vi "Calibration.vi"   [LabVIEW 2013]
uses:
  Global Variables.vi
  Global Refnums.vi
types:
  T1 = typedef "WPI_AnalogChannelDevRef.ctl" = cluster{"DevStatus":errorcluster, "Analog Module":T2, "Analog Channel":T3}
  T2 = typedef "FPGA_TypedefAnalogModule.ctl" = enum16{"Analog Module 1", "Analog Module 2"}
  T3 = typedef "FPGA_AIChannel.ctl" = enum8{"AI 1", "AI 2", "AI 3", "AI 4", "AI 5", "AI 6", "AI 7", "AI 8", "Invalid"}
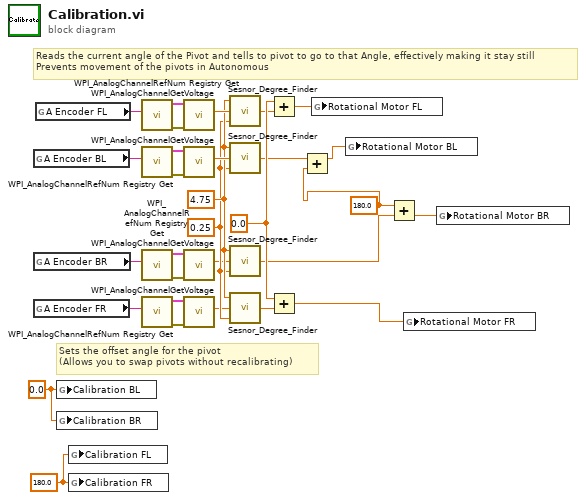
[diagram p0: block diagram]
diagram:
  w1 = 180.0 ("x")
  w22 = 0.0
  w8 = 0.25
  w9 = 4.75
  w29 = 0.0
  w30 = 180.0
  # "Sets the offset angle for the pivot\n(Allows you to swap pivots without recalibrating)"
  # "Reads the current angle of the Pivot and tells to pivot to go to that Angle, effectively making it stay still\nPrevents movement of the pivots in Autonomous"
  n1 = global read "Global Refnums.vi" "A Encoder BL"() -> (w28:string)
  n2 = global read "Global Refnums.vi" "A Encoder BR"() -> (w27:string)
  n3 = global read "Global Refnums.vi" "A Encoder FR"() -> (w25:string)
  n4 = global read "Global Refnums.vi" "A Encoder FL"() -> (w26:string)
  n5 = global write "Global Variables.vi" "Calibration BL"(w29) -> ()
  n6 = global write "Global Variables.vi" "Calibration BR"(w29) -> ()
  n7 = global write "Global Variables.vi" "Calibration FL"(w30) -> ()
  n8 = global write "Global Variables.vi" "Calibration FR"(w30) -> ()
  n9 = call <vilib>:"WPI_AnalogChannelRefNum Registry Get.vi"("refnum name"=w26) -> ("error out"=w17:errorcluster, "AIDeviceRef"=w16:T1)  [unwired: 9 in]
  n10 = call <vilib>:"WPI_AnalogChannelRefNum Registry Get.vi"("refnum name"=w28) -> ("error out"=w20:errorcluster, "AIDeviceRef"=w21:T1)  [unwired: 9 in]
  n11 = call <vilib>:"WPI_AnalogChannelRefNum Registry Get.vi"("refnum name"=w27) -> ("error out"=w19:errorcluster, "AIDeviceRef"=w18:T1)  [unwired: 9 in]
  n12 = call <vilib>:"WPI_AnalogChannelRefNum Registry Get.vi"("refnum name"=w25) -> ("error out"=w15:errorcluster, "AIDeviceRef"=w14:T1)  [unwired: 9 in]
  n13 = call <vilib>:"WPI_AnalogChannelGetVoltage.vi"("error in (no error)"=w17, "AIDeviceRef"=w16) -> ("Voltage"=w12:dbl)  [unwired: 7 in, 2 out]
  n14 = call <vilib>:"WPI_AnalogChannelGetVoltage.vi"("error in (no error)"=w20, "AIDeviceRef"=w21) -> ("Voltage"=w11:dbl)  [unwired: 7 in, 2 out]
  n15 = call <vilib>:"WPI_AnalogChannelGetVoltage.vi"("error in (no error)"=w19, "AIDeviceRef"=w18) -> ("Voltage"=w7:dbl)  [unwired: 7 in, 2 out]
  n16 = call <vilib>:"WPI_AnalogChannelGetVoltage.vi"("error in (no error)"=w15, "AIDeviceRef"=w14) -> ("Voltage"=w6:dbl)  [unwired: 7 in, 2 out]
  n17 = call "Sesnor_Degree_Finder.vi"("Minimum Volts"=w8, "Voltage"=w12, "Max Volts"=w9) -> ("Degrees"=w13:dbl)
  n18 = call "Sesnor_Degree_Finder.vi"("Minimum Volts"=w8, "Voltage"=w11, "Max Volts"=w9) -> ("Degrees"=w10:dbl)
  n19 = call "Sesnor_Degree_Finder.vi"("Minimum Volts"=w8, "Voltage"=w7, "Max Volts"=w9) -> ("Degrees"=w5:dbl)
  n20 = call "Sesnor_Degree_Finder.vi"("Minimum Volts"=w8, "Voltage"=w6, "Max Volts"=w9) -> ("Degrees"=w4:dbl)
  n21 = Add(x=w22, y=w13) -> (x+y=w24:dbl)
  n22 = Add(x=w22, y=w4) -> (x+y=w23:dbl)
  n23 = Add(x=w10, y=w1) -> (x+y=w2:dbl)
  n24 = global write "Global Variables.vi" "Rotational Motor FL"(w24) -> ()
  n25 = global write "Global Variables.vi" "Rotational Motor BL"(w2) -> ()
  n26 = Add(x=w1, y=w5) -> (x+y=w3:dbl)
  n27 = global write "Global Variables.vi" "Rotational Motor FR"(w23) -> ()
  n28 = global write "Global Variables.vi" "Rotational Motor BR"(w3) -> ()
